vi "柱塞泵KB写入.vi"(7 "是否启用通讯通知":bool, 8 "error in (no error)":errorcluster, 9 "B":sgl, 10 "K":sgl, 11 "Slave ID":T1) -> (0 "error out":errorcluster)   [LabVIEW 2016, in "质控单元V1.lvlib"]
uses:
  <vilib>/Plasmionique/MB Master/MB_Master/MB_Master.lvclass
  <vilib>/Plasmionique/MB Master/MB Master.lvlib
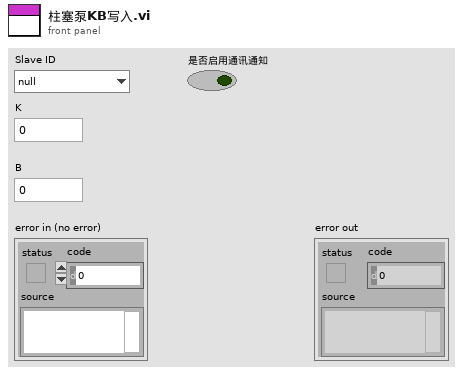
[diagram p1: front panel]
types:
  T1 = typedef "质控单元V1.lvlib/质控slave id.ctl" = enum16{"null", "氨氮", "总磷", "CODMn", "CODCr", "总氮"}
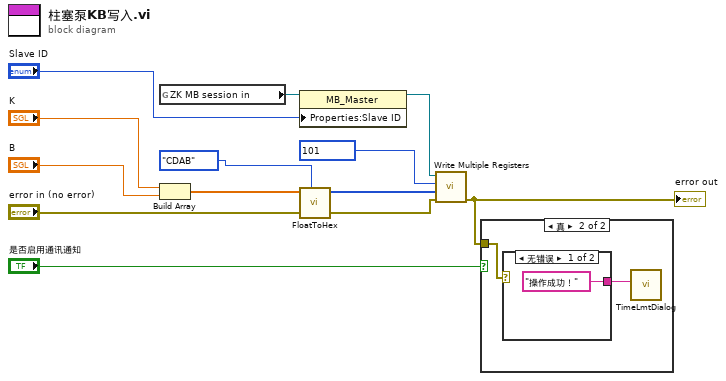
[diagram p0: block diagram]
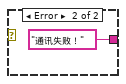
[diagram p3: hidden frame]
diagram:
  n1 = global read "ZK非断电保存全局变量.vi" "ZK MB session in"() -> (w11:refnum<class "MB_Master.lvclass">)
  n2 = Build Array("K", "B") -> (w6:sgl[])
  n3 = property class="MB_Master"(reference=w11, "Properties:Slave ID"="Slave ID") -> (reference out=w9:refnum<class "MB_Master.lvclass">)  [unwired: 1 in, 1 out]
  n4 = call "FloatToHex.vi"("转换类型"=enum16{"DCBA", "CDAB"}."CDAB", "浮点数"=w6) -> ("CDAB整形输出"=w5:u16[])  [unwired: 9 in]
  n5 = call <vilib>:"Write Multiple Registers.vi"("error in (no error)"="error in (no error)", "values"=w5, "starting address"=u16 101, "MB session in"=w9) -> ("error out"=w3:errorcluster)  [unwired: 6 in, 1 out]
  "error out" <- w3
  n6 = case shown="真" "是否启用通讯通知" {
    tunnel: w3 -> [_ w14]
    frame False {
    }
    frame True {
      n7 = case shown="无错误" w14 {
        tunnel: ["操作成功！" "通讯失败！"] -> w13
        frame No Error {
        }
        frame Error {
        }
      }
      n8 = call "TimeLmtDialog.vi"("Infoin"=w13) -> ()  [unwired: 11 in]
    }
  }
